vi "Read Excel Values_LV2012_NI Verified.vi"() -> (2 "ExcelData":string[][](array[string]))   [LabVIEW 2017]
doc: "This simple program is a demonstration of how to use the LabVIEW Report Generation Toolkit to read data from Excel."
uses:
  <vilib>/addons/_office/excel.llb/Excel Get Data ([str]).vi
  <vilib>/Utility/NIReport.llb/NI_report.lvclass
  <vilib>/Utility/NIReport.llb/Excel/NI_Excel.lvclass
  <vilib>/addons/_office/NI_ReportGenerationToolkit.lvlib
panel:
  in  "start path":path=path ""
  out "size(s)":i32[](array[numeric])
  # "Overview: This simple program is a demonstration of how to use the LabVIEW Report Generation Toolkit to read data from Excel.\nRequirements: LabVIEW 2012 (or compatible), LabVIEW Report Generation Toolkit 2012 (or compatible)\nInstructions:\n1. Run the VI\n2. You will be prompted to enter the location for the excel file, browse for the the excel file located in the same directory of this VI\n3. Click OK"
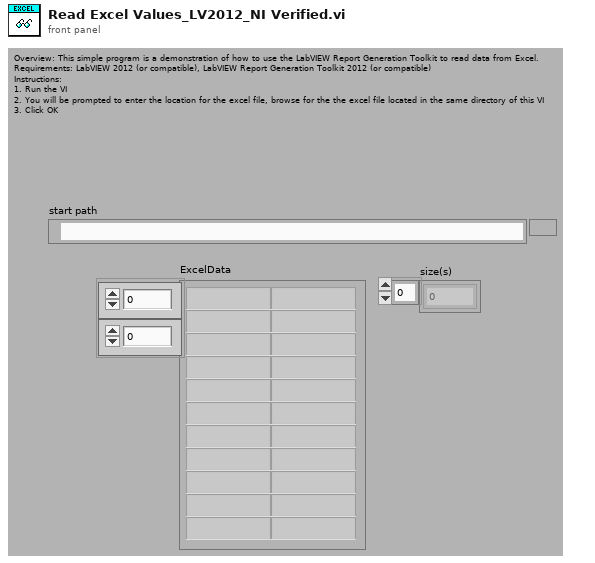
[diagram p1: front panel]
types:
  T1 = enum16{"Standard Report", "HTML", "Word", "Excel"}
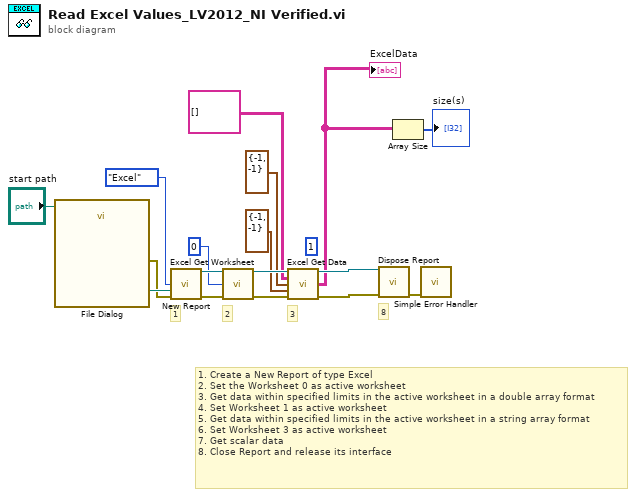
[diagram p0: block diagram]
diagram:
  (unwired) 1 ("worksheet index (0)")
  # "1. Create a New Report of type Excel\n2. Set the Worksheet 0 as active worksheet\n3. Get data within specified limits in the active worksheet in a double array format\n4. Set Worksheet 1 as active worksheet\n5. Get data within specified limits in the active worksheet in a string array format \n6. Set Worksheet 3 as active worksheet\n7. Get scalar data \n8. Close Report and release its interface"
  # "8"
  # "3"
  # "2"
  # "1"
  n1 = call "File Dialog"("start path"="start path") -> ("selected path"=w8:path, "error out"=w7:errorcluster)  [unwired: 6 in, 7 out]
  n2 = call <vilib>:"New Report.vi"("report type"=T1."Excel", "template (empty)"=w8, "error in (no error)"=w7) -> ("report out"=w17:refnum<class "NI_report.lvclass">, "error out"=w13:errorcluster)  [unwired: 3 in, 8 out]
  n3 = call <vilib>:"Excel Get Worksheet.vi"("report in"=w17, "worksheet index (0)"=0, "error in (no error)"=w13) -> ("report out"=w16:refnum<class "NI_report.lvclass">, "error out"=w12:errorcluster)  [unwired: 11 out]
  n4 = call-poly <vilib>:"Excel Get Data.vi"("report in"=w16, "data type"=string[][] [], "start (-1, -1)"=cluster{"row":i32, "column":i32} {"row"=-1, "column"=-1}, "end (-1, -1)"=cluster{"row":i32, "column":i32} {"row"=-1, "column"=-1}, "error in (no error)"=w12) -> ("report out"=w4:refnum<class "NI_report.lvclass">, "data"=w3:string[][], "error out"=w5:errorcluster)  [unwired: 8 out]
  "ExcelData" <- w3
  n5 = call-dynamic "Dispose Report.vi"("report in"=w4, "error in (no error)"=w5) -> ("error out"=w9:errorcluster)  [unwired: 3 in, 10 out]
  n6 = Array Size(array=w3) -> (size(s)=→"size(s)":i32[])
  n7 = call <vilib>:"Simple Error Handler.vi"("error in (no error)"=w9) -> ()  [unwired: 4 in, 5 out]
